vi "Material-ConfigDialog-BroadcastMessage.vi"(0 "Configuration Dialog":refnum<class "Material-ConfigDialog.lvclass">, 5 "Parameter":string, 7 "Payload":variant, 11 "error in":errorcluster) -> (4 "Configuration Dialog out":refnum<class "Material-ConfigDialog.lvclass">, 15 "error out":errorcluster)   [LabVIEW 2013, in "Material-ConfigDialog.lvclass"]
uses:
  Material-ConfigDialog.lvclass
  Reuse Library/featherweight/Core/Messaging/Messenger.Actor/FTW-Messenger-Actor.lvclass
panel:
  # "Inputs"
  # "Outputs"
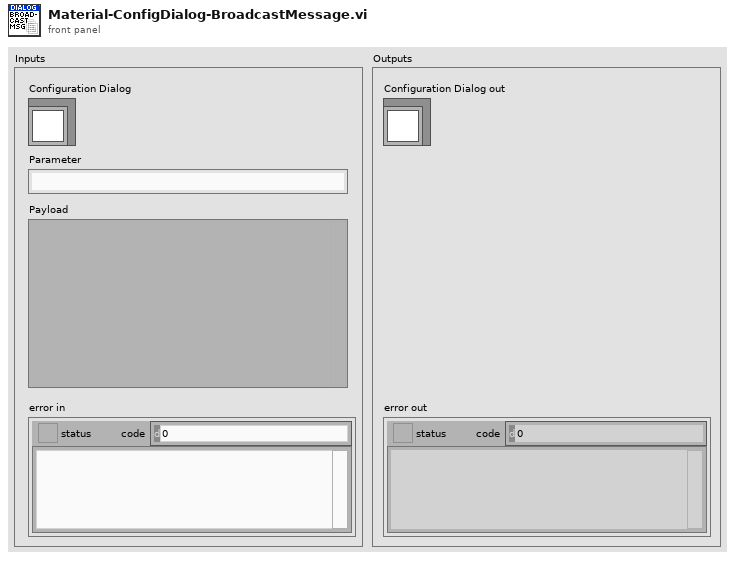
[diagram p1: front panel]
types:
  T1 = typedef "Material-ConfigDialog.lvclass/Material-ConfigDialog-Page.ctl" = cluster{"Initialized?":bool, "PageID":string, "Messenger":refnum<class "FTW-Messenger-Actor.lvclass">}
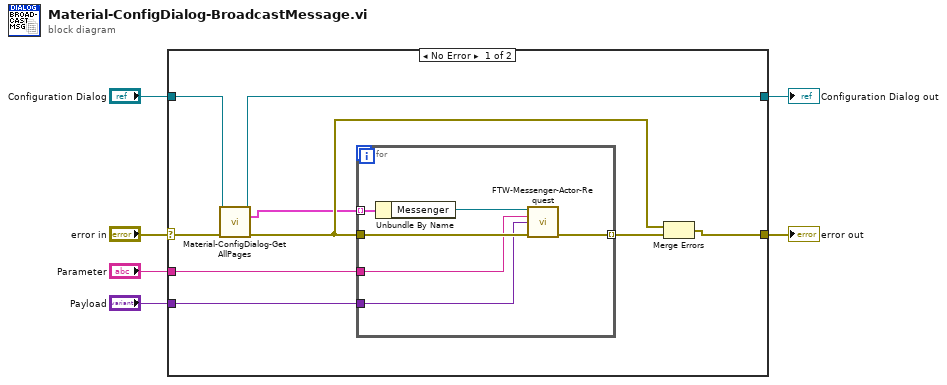
[diagram p0: block diagram]
diagram:
  n1 = case shown="No Error" "error in" {
    selector: "error in" -> [w9 w23]
    tunnel: [w12 w23] -> w6
    tunnel: [w10 w22] -> w4
    tunnel: "Configuration Dialog" -> [w11 w22]
    tunnel: "Parameter" -> [w15 _]
    tunnel: "Payload" -> [w14 _]
    frame No Error {
      n2 = call "Material-ConfigDialog-GetAllPages.vi"("Configuration Dialog"=w11, "error in"=w9) -> ("Configuration Dialog out"=w10:refnum<class "Material-ConfigDialog.lvclass">, "Pages"=w7:T1[], "error out"=w8:errorcluster)  [unwired: 11 in]
      n3 = for {
        tunnel: w7 -> [w21] mode=indexing
        tunnel: w15 -> [w18]
        tunnel: w14 -> [w17]
        tunnel: w8 -> [w19]
        tunnel: [w16] -> w13 mode=indexing
        n4 = Unbundle By Name(w21) -> ("Messenger"=w20:refnum<class "FTW-Messenger-Actor.lvclass">)
        n5 = call-dynamic "FTW-Messenger-Actor-Request.vi"("Messenger"=w20, "Parameter"=w18, "Payload"=w17, "error in"=w19) -> ("error out"=w16:errorcluster)  [unwired: 10 in, 1 out]
      }
      n6 = Merge Errors(w8, w13) -> (w12:errorcluster)
    }
    frame Error {
    }
  }
  "error out" <- w6
  "Configuration Dialog out" <- w4
